vi "Test 3010.vi"() -> ()   [LabVIEW 2014]
uses:
  3010.lvclass
  <vilib>/Utility/file.llb/Write To Spreadsheet File (DBL).vi
panel:
  out "Temperature":T1
  out "Status":T2
  out "Buffer":cluster{"6 s":u32, "1 s":u32}
  out "dataOut":dbl(graph)
  in  "Port":refnum<visa-resource-name>="COM6"
  out "time":timestamp format="%<%H:%M:%S%2u>T"
  out "error out":errorcluster
  out "dispConc":sgl
  out "counts":u32
  out "time":u32
  in  "stop":bool
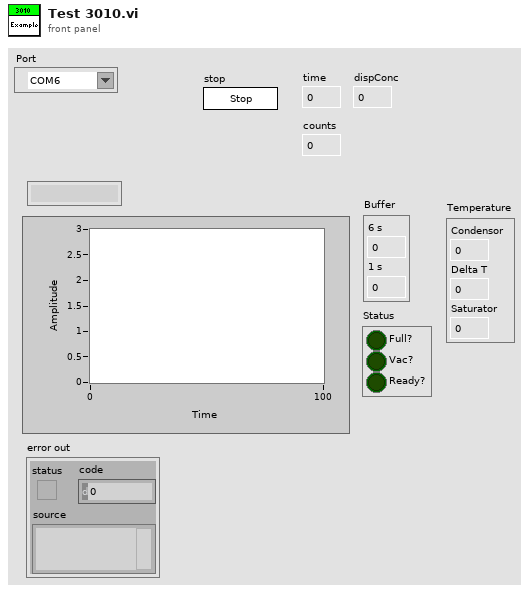
[diagram p1: front panel]
types:
  T1 = cluster{"Condensor":sgl, "Delta T":sgl, "Saturator":sgl}
  T2 = cluster{"Full?":bool, "Vac?":bool, "Ready?":bool}
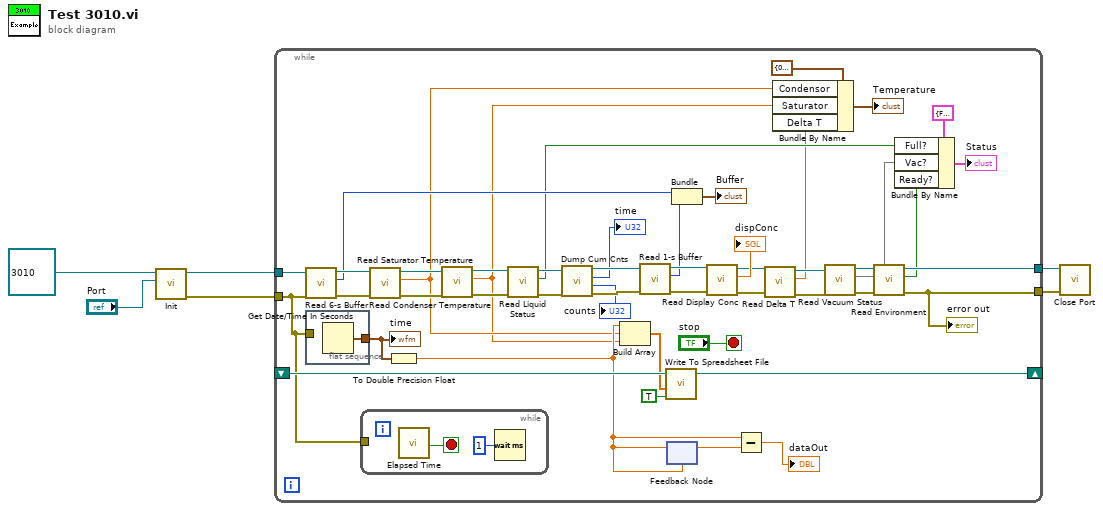
[diagram p0: block diagram]
diagram:
  n1 = call-dynamic "Init.vi"("Port"="Port", "3010 in"=refnum<class "3010.lvclass"> refnum ("3010.lvclass")) -> ("error out"=w4:errorcluster, "3010 out"=w3:refnum<class "3010.lvclass">)  [unwired: 8 in]
  n2 = while {
    tunnel: w4 -> [w20]
    tunnel: w3 -> [w53]
    tunnel: [w40] -> w2
    tunnel: [w39] -> w1
    shift-right: [w38] -> _
    shift-left: _ -> [w37]
    stop <- "stop" stop-if-true
    n3 = call "Read 6-s Buffer.vi"("error in"=w20, "3010 in"=w53) -> ("error out"=w51:errorcluster, "6_s Buffer"=w18:u32, "3010 out"=w52:refnum<class "3010.lvclass">)  [unwired: 7 in]
    n4 = flat-sequence {
      tunnel: w20 -> [_]
      tunnel: [w56] -> w36
      frame #0 {
        n5 = Get Date/Time In Seconds() -> (seconds since 1Jan1904=w56:timestamp)
      }
    }
    n6 = while {
      tunnel: w20 -> [_]
      stop <- w55 stop-if-true
      n7 = call "Elapsed Time"() -> ("Time has Elapsed"=w55:bool)  [unwired: 12 in, 7 out]
      n8 = Wait (ms)(milliseconds to wait=u32 1) -> ()  [unwired: 1 out]
    }
    n9 = call "Read Condenser Temperature.vi"("error in"=w51, "3010 in"=w52) -> ("error out"=w49:errorcluster, "condT"=w10:sgl, "3010 out"=w50:refnum<class "3010.lvclass">)  [unwired: 7 in]
    n10 = To Double Precision Float(number=w36) -> (double precision float=w33:dbl)
    n11 = call "Read Saturator Temperature.vi"("error in"=w49, "3010 in"=w50) -> ("error out"=w47:errorcluster, "satT"=w9:sgl, "3010 out"=w48:refnum<class "3010.lvclass">)  [unwired: 7 in]
    n12 = call "Read Liquid Status.vi"("error in"=w47, "3010 in"=w48) -> ("error out"=w30:errorcluster, "Full?"=w15:bool, "3010 out"=w31:refnum<class "3010.lvclass">)  [unwired: 7 in]
    n13 = call "Dump Cum Cnts.vi"("error in"=w30, "3010 in"=w31) -> ("error out"=w45:errorcluster, "counts"=→"counts":u32, "time"=→"time":u32, "3010 out"=w46:refnum<class "3010.lvclass">)  [unwired: 6 in]
    n14 = Build Array(w33, w10, w9) -> (w35:dbl[])
    n15 = call "Read 1-s Buffer.vi"("error in"=w45, "3010 in"=w46) -> ("error out"=w27:errorcluster, "1_s Buffer"=w19:u32, "3010 out"=w28:refnum<class "3010.lvclass">)  [unwired: 7 in]
    n16 = call-poly <vilib>:"Write To Spreadsheet File.vi"("append to file? (new file:F)"=TRUE, "1D data"=w35, "file path (dialog if empty)"=w37) -> ("new file path (Not A Path if cancelled)"=w38:path)  [unwired: 5 in]
    n17 = feedback-in #1(w33) -> ()
    n18 = feedback #1(w33) -> (w32:dbl)
    n19 = Bundle("6_s Buffer"=w18, "1_s Buffer"=w19) -> (→"Buffer":cluster{"6_s Buffer":u32, "1_s Buffer":u32})  [unwired: 1 in]
    n20 = call "Read Display Conc.vi"("error in"=w27, "3010 in"=w28) -> ("error out"=w25:errorcluster, "dispConc"=→"dispConc":sgl, "3010 out"=w26:refnum<class "3010.lvclass">)  [unwired: 7 in]
    n21 = Subtract(x=w33, y=w32) -> (x-y=→"dataOut":dbl)
    n22 = call "Read Delta T.vi"("error in (no error)"=w25, "3010 in"=w26) -> ("error out"=w21:errorcluster, "dT"=w8:dbl, "3010 out"=w22:refnum<class "3010.lvclass">)  [unwired: 7 in]
    n23 = Bundle By Name(cluster=T1 {"Condensor"=0.0, "Delta T"=0.0, "Saturator"=0.0} ("Temperature"), "Condensor"=w10, "Saturator"=w9, "Delta T"=w8) -> (→"Temperature":T1)
    n24 = call "Read Vacuum Status.vi"("error in (no error)"=w21, "3010 in"=w22) -> ("error out"=w23:errorcluster, 2:w14, "3010 out"=w24:refnum<class "3010.lvclass">)  [unwired: 7 in]
    n25 = call "Read Environment.vi"("error in"=w23, "3010 in"=w24) -> ("error out"=w39:errorcluster, "Ready?"=w13:bool, "3010 out"=w40:refnum<class "3010.lvclass">)  [unwired: 7 in]
    "error out" <- w39
    n26 = Bundle By Name(cluster=T2 {"Full?"=FALSE, "Vac?"=FALSE, "Ready?"=FALSE} ("Status"), "Full?"=w15, "Vac?"=w14, "Ready?"=w13) -> (→"Status":T2)
    "time" <- w36
  }
  n27 = call-dynamic "Close Port.vi"("error in (no error)"=w1, "Serial IO in"=w2) -> ()  [unwired: 8 in, 2 out]
